vi "StateExample_copy.vi"() -> ()   [LabVIEW 2014]
panel:
  out "samples per acquisition":dbl
  out "sampling rate":dbl
  out "login status":bool
  in  "Stop Button":bool
  in  "Menu cluster":T1
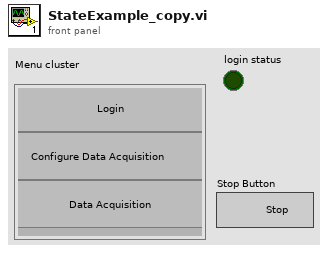
[diagram p1: front panel]
types:
  T1 = cluster{"Configuration":bool, "Configuration 2":bool, "Configuration 3":bool}
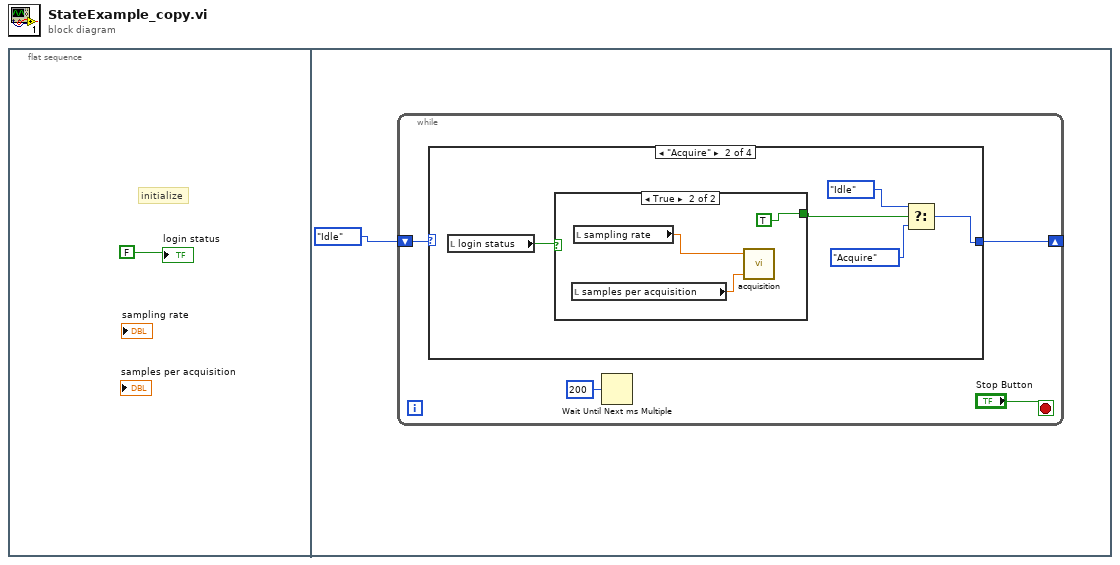
[diagram p0: block diagram]
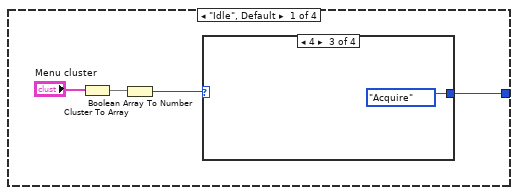
[diagram p2: hidden frame]
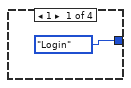
[diagram p3: hidden frame]
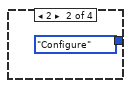
[diagram p4: hidden frame]
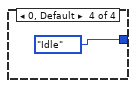
[diagram p5: hidden frame]
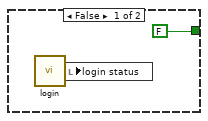
[diagram p6: hidden frame]
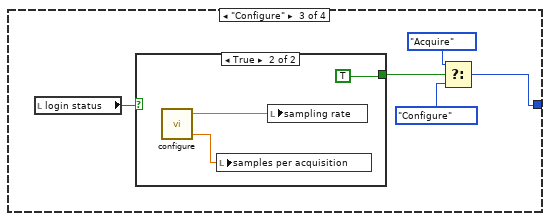
[diagram p7: hidden frame]
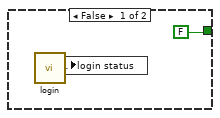
[diagram p8: hidden frame]
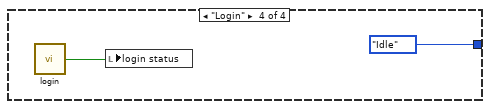
[diagram p9: hidden frame]
diagram:
  n1 = flat-sequence {
    frame #0 {
      # "initialize"
      "login status" <- FALSE
    }
    frame #1 {
      n2 = while {
        shift-right: [w4] -> _
        shift-left: enum16{"Idle", "Acquire", "Configure", "Login"}."Idle" -> [w5]
        stop <- "Stop Button" stop-if-true
        n3 = case shown="\"Acquire\"" w5 {
          tunnel: [w7 w15 w26 enum16{"Idle", "Acquire", "Configure", "Login"}."Idle"] -> w4
          frame "Idle", Default {
            n4 = Cluster To Array(cluster="Menu cluster") -> (array=w9:bool[])
            n5 = Boolean Array To Number(Boolean array=w9) -> (number=w8:u32)
            n6 = case shown="4" w8 {
              tunnel: [enum16{"Idle", "Acquire", "Configure", "Login"}."Login" enum16{"Idle", "Acquire", "Configure", "Login"}."Configure" enum16{"Idle", "Acquire", "Configure", "Login"}."Acquire" enum16{"Idle", "Acquire", "Configure", "Login"}."Idle"] -> w7
              frame 1 {
              }
              frame 2 {
              }
              frame 4 {
              }
              frame 0, Default {
              }
            }
          }
          frame "Acquire" {
            n7 = local read "login status"() -> (w19:bool)
            n8 = case shown="True" w19 {
              tunnel: [FALSE TRUE] -> w18
              frame False {
                n9 = call "login.vi"() -> ("Corret"=w21:bool)  [unwired: 1 in]
                n10 = local write "login status"(w21) -> ()
              }
              frame True {
                n11 = local read "samples per acquisition"() -> (w22:dbl)
                n12 = local read "sampling rate"() -> (w23:dbl)
                n13 = call "acquisition.vi"("samples per acquisition"=w22, "sampling rate"=w23) -> ()  [unwired: 2 in]
              }
            }
            n14 = Select(t=enum16{"Idle", "Acquire", "Configure", "Login"}."Idle", s=w18, f=enum16{"Idle", "Acquire", "Configure", "Login"}."Acquire") -> (s? t:f=w15:enum16{"Idle", "Acquire", "Configure", "Login"})
          }
          frame "Configure" {
            n15 = local read "login status"() -> (w29:bool)
            n16 = case shown="True" w29 {
              tunnel: [FALSE TRUE] -> w28
              frame False {
                n17 = call "login.vi"() -> ("Corret"=w31:bool)  [unwired: 1 in]
                n18 = local write "login status"(w31) -> ()
              }
              frame True {
                n19 = call "configure.vi"() -> ("show samples per acquisition"=w32:dbl, "show sampling rate (samples/sec)"=w33:dbl)  [unwired: 4 in]
                n20 = local write "samples per acquisition"(w32) -> ()
                n21 = local write "sampling rate"(w33) -> ()
              }
            }
            n22 = Select(t=enum16{"Idle", "Acquire", "Configure", "Login"}."Acquire", s=w28, f=enum16{"Idle", "Acquire", "Configure", "Login"}."Configure") -> (s? t:f=w26:enum16{"Idle", "Acquire", "Configure", "Login"})
          }
          frame "Login" {
            n23 = call "login.vi"() -> ("Corret"=w35:bool)  [unwired: 1 in]
            n24 = local write "login status"(w35) -> ()
          }
        }
        n25 = Wait Until Next ms Multiple(millisecond multiple=u32 200) -> ()  [unwired: 1 out]
      }
    }
  }
